vi "8500_ShortEnable.vi"() -> ()   [LabVIEW 2017]
uses:
  <instrlib>/BK Precision 85XX Series/BK Precision 85XX Series.lvlib
panel:
  out "error out":errorcluster
  out "Terminal Input Power (10)":dbl(knob) scale=0.0..10.0 scale format="%#_3f"
  out "Terminal Input Current (A)":dbl(knob) scale=0.0..10.0 scale format="%#_3g"
  out "Terminal Input Voltage (V)":dbl(knob) scale=0.0..10.0 scale format="%#_3g"
  in  "Enable Input Terminals (F: Off)":bool
  in  "VISA resource name":refnum<visa-resource-name>
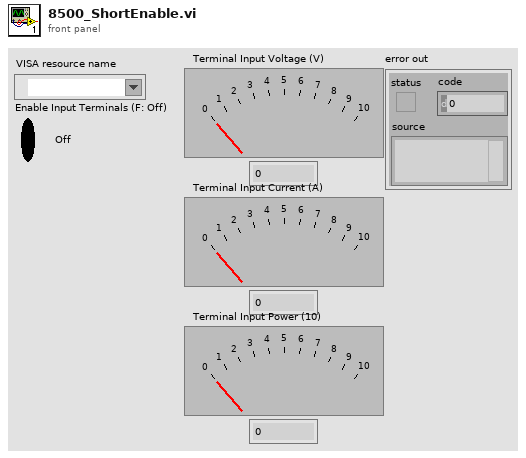
[diagram p1: front panel]
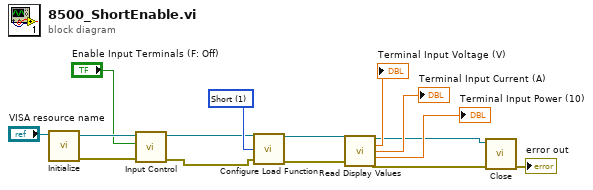
[diagram p0: block diagram]
diagram:
  w15 = u16 1 items=["Fixed", "Short", "Transient", "List", "Battery"] ("Function (0:FIXED)")
  n1 = call <instrlib>:"Initialize.vi"("VISA resource name"="VISA resource name") -> ("error out"=w12:errorcluster, "VISA resource name out"=w13:refnum<visa-resource-name>)  [unwired: 9 in]
  n2 = call <instrlib>:"Input Control.vi"("error in (no error)"=w12, "Enable Input Terminals (F: Off)"="Enable Input Terminals (F: Off)", "VISA resource name"=w13) -> ("error out"=w9:errorcluster, "VISA resource name out"=w10:refnum<visa-resource-name>)  [unwired: 7 in]
  n3 = call <instrlib>:"Configure Load Function.vi"("VISA resource name"=w10, "Function (0:FIXED)"=w15, "error in (no error)"=w9) -> ("VISA resource name out"=w8:refnum<visa-resource-name>, "error out"=w7:errorcluster)  [unwired: 11 in]
  n4 = call <instrlib>:"Read Display Values.vi"("VISA resource name"=w8, "error in (no error)"=w7) -> ("VISA resource name out"=w3:refnum<visa-resource-name>, "Terminal Input Voltage (V)"=→"Terminal Input Voltage (V)":dbl, "Terminal Input Current (A)"=→"Terminal Input Current (A)":dbl, "Terminal Input Power (W)"=→"Terminal Input Power (10)":dbl, "error out"=w2:errorcluster)  [unwired: 9 in]
  n5 = call <instrlib>:"Close.vi"("error in (no error)"=w2, "VISA resource name"=w3) -> ("error out"=→"error out":errorcluster)  [unwired: 9 in]
